vi "Read Device List.vi"(8 "error in":errorcluster, 11 "Config in":refnum<class "Config.lvclass">) -> (0 "error out":errorcluster, 2 "Device List":string[](array[string]), 3 "Config out":refnum<class "Config.lvclass">)   [LabVIEW 2023, in "Config.lvlib" / "Config.lvclass"]
uses:
  Config.lvclass
  Config.lvclass/Config.ctl
  <vilib>/Utility/config.llb/NI_LVConfig.lvlib
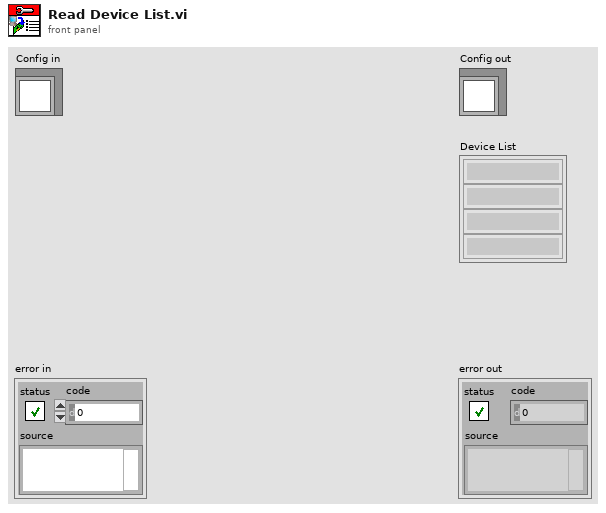
[diagram p1: front panel]
types:
  T1 = typedef "NI_LVConfig.lvlib/Config Data RefNum.ctl" = refnum<k1>
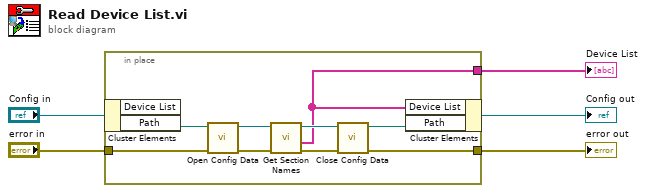
[diagram p0: block diagram]
diagram:
  n1 = in-place {
    in-place-border: "error in" -> [w8]
    in-place-border: [w7] -> w2
    in-place-border: [w6] -> w1
    n2 = in-place-cluster #1("Config in") -> ("Path"=w14:path)  [unwired: 1 out]
    n3 = call <vilib>:"Open Config Data.vi"("error in (no error)"=w8, "configuration file path"=w14) -> ("error out"=w12:errorcluster, "refnum"=w13:T1)  [unwired: 7 in, 1 out]
    n4 = call <vilib>:"Get Section Names.vi"("error in (no error)"=w12, "refnum"=w13) -> ("error out"=w10:errorcluster, "section names"=w6:string[], "refnum out"=w11:T1)  [unwired: 7 in]
    n5 = call <vilib>:"Close Config Data.vi"("error in (no error)"=w10, "refnum"=w11) -> ("error out"=w7:errorcluster, "file path"=w9:path)  [unwired: 8 in]
    n6 = in-place-cluster #1("Device List"=w6, "Path"=w9) -> (→"Config out":refnum<class "Config.lvclass">)
  }
  "error out" <- w2
  "Device List" <- w1
